vi "Counter with Race Condition.vi"() -> ()   [LabVIEW 2012]
panel:
  out "Running Total":i32
  in  "Stop Button":bool
  out "Loop Count Difference":i32
  out "Loop Count 2":i32
  out "Loop Count 1":i32
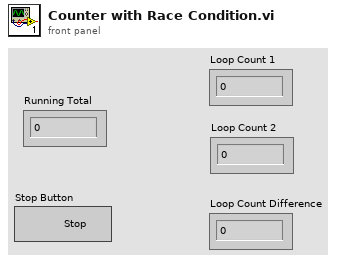
[diagram p1: front panel]
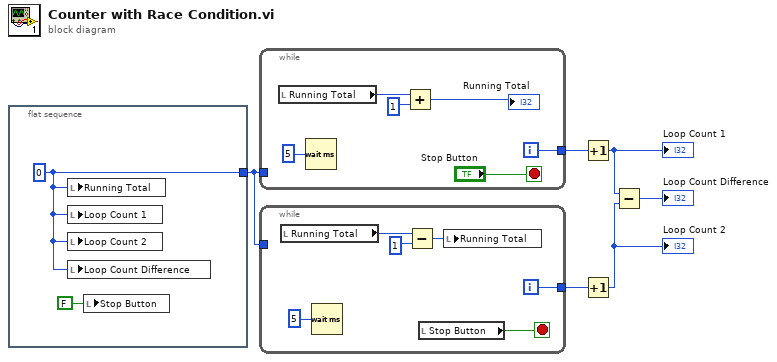
[diagram p0: block diagram]
diagram:
  n1 = flat-sequence {
    tunnel: [w7] -> w4
    frame #0 {
      w7 = 0 ("Running Total")
      n2 = local write "Running Total"(w7) -> ()
      n3 = local write "Loop Count 1"(w7) -> ()
      n4 = local write "Loop Count 2"(w7) -> ()
      n5 = local write "Loop Count Difference"(w7) -> ()
      n6 = local write "Stop Button"(FALSE ("Stop Button")) -> ()
    }
  }
  n7 = while {
    tunnel: [w10] -> w6
    tunnel: w4 -> [_]
    i -> [w10]
    stop <- "Stop Button" stop-if-true
    n8 = local read "Running Total"() -> (w11:i32)
    n9 = Wait (ms)(milliseconds to wait=u32 5) -> ()  [unwired: 1 out]
    n10 = Add(x=w11, y=1 ("x")) -> (x+y=→"Running Total":i32)
  }
  n11 = while {
    tunnel: [w18] -> w5
    tunnel: w4 -> [_]
    i -> [w18]
    stop <- w20 stop-if-true
    n12 = local read "Running Total"() -> (w17:i32)
    n13 = Wait (ms)(milliseconds to wait=u32 5) -> ()  [unwired: 1 out]
    n14 = Subtract(x=w17, y=1 ("x")) -> (x-y=w15:i32)
    n15 = local read "Stop Button"() -> (w20:bool)
    n16 = local write "Running Total"(w15) -> ()
  }
  n17 = Increment(x=w6) -> (x+1=w3:i32)
  "Loop Count 1" <- w3
  n18 = Increment(x=w5) -> (x+1=w2:i32)
  "Loop Count 2" <- w2
  n19 = Subtract(x=w3, y=w2) -> (x-y=→"Loop Count Difference":i32)
